vi "loop_timeout.vi"   [LabVIEW 2015]
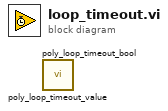
[diagram p0: block diagram]
diagram:
  n1 = call "poly_loop_timeout_value.vi"() -> ()  [unwired: 7 in, 1 out]
  n2 = call "poly_loop_timeout_bool.vi"() -> ()  [unwired: 7 in, 1 out]
